vi "9.2.vi"() -> ()   [LabVIEW 2020]
panel:
  in  "y 3":i32
  in  "y 2":i32
  out "ScanCode":i16
  out "Waveform Graph":cluster{i32, i32, dbl[]}(graph)
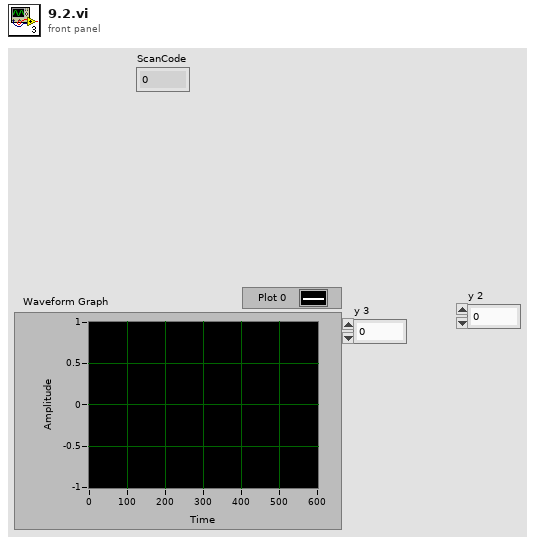
[diagram p1: front panel]
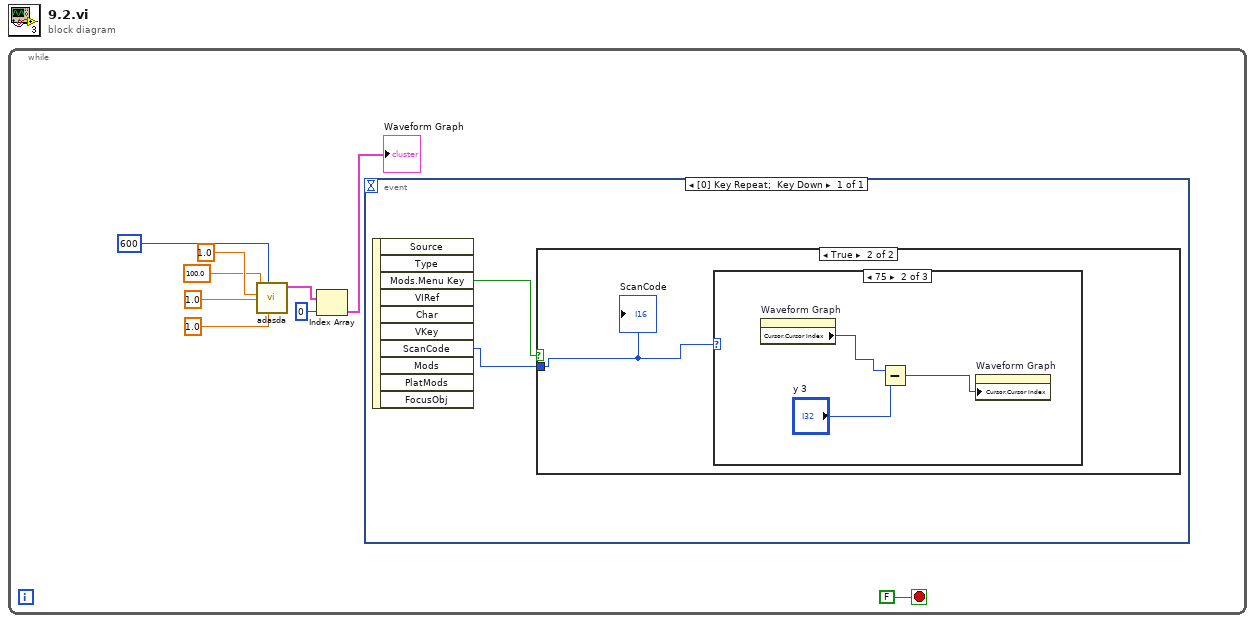
[diagram p0: block diagram]
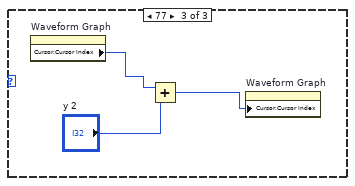
[diagram p4: hidden frame]
diagram:
  n1 = while {
    stop <- FALSE stop-if-true
    n2 = call "adasda.vi"("cos amp"=1.0, "Puntkide arv"=600, "sin amp"=1.0, "cos sagedus"=1.0, "sin sagedus"=100.0) -> ("appended array"=w1:cluster{i32, i32, dbl[]}[])  [unwired: 5 in, 1 out]
    n3 = Index Array(array=w1, index=0) -> (element=→"Waveform Graph":cluster{i32, i32, dbl[]})
    n4 = event shown="[0] Key Repeat;  Key Down" {
      selector: _ -> [_]
      dyn-events: _ -> [_]
      timeout: _ -> [_]
      event Key Repeat; Key Down {
        n5 = event-data() -> ("Mods.Menu Key"=w11:bool, "ScanCode"=w10:i16)  [unwired: 1 in, 8 out]
        n6 = case shown="True" w11 {
          tunnel: w10 -> [_ w12]
          frame False {
          }
          frame True {
            n7 = case shown="75" w12 {
              frame 0, Default {
              }
              frame 75 {
                n8 = property on="Waveform Graph" class="WFGraph (strict)"() -> ("Cursor.Cursor Index"=w14:i32)  [unwired: 2 in, 2 out]
                n9 = Subtract(x=w14, y="y 3") -> (x-y=w13:i32)
                n10 = property on="Waveform Graph" class="WFGraph (strict)"("Cursor.Cursor Index"=w13) -> ()  [unwired: 2 in, 2 out]
              }
              frame 77 {
                n11 = property on="Waveform Graph" class="WFGraph (strict)"() -> ("Cursor.Cursor Index"=w17:i32)  [unwired: 2 in, 2 out]
                n12 = Add(x=w17, y="y 2") -> (x+y=w16:i32)
                n13 = property on="Waveform Graph" class="WFGraph (strict)"("Cursor.Cursor Index"=w16) -> ()  [unwired: 2 in, 2 out]
              }
            }
            "ScanCode" <- w12
          }
        }
      }
    }
  }
